vi "网分校准.vi"(8 "error in (no error)":errorcluster, 11 "keysight in":refnum<class "keysight.lvclass">) -> (0 "error out":errorcluster, 3 "keysight out":refnum<class "keysight.lvclass">)   [LabVIEW 2015, in "keysight.lvclass"]
uses:
  keysight.lvclass
  network_Global/Global.vi
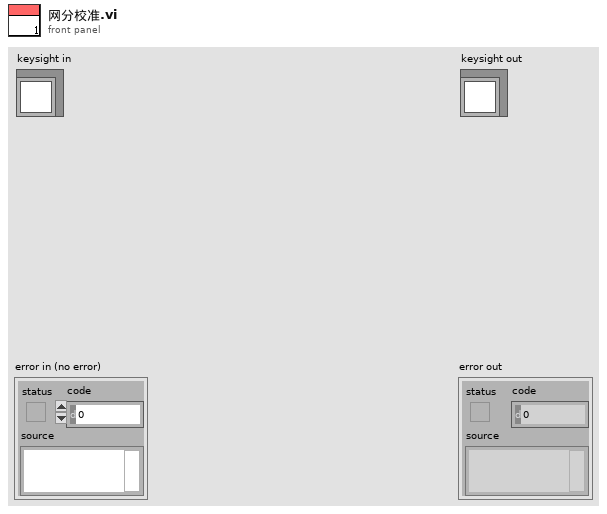
[diagram p1: front panel]
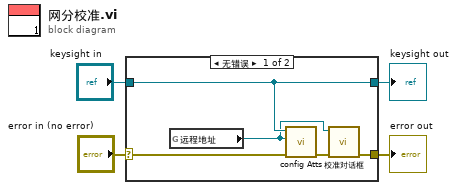
[diagram p0: block diagram]
diagram:
  n1 = case shown="无错误" "error in (no error)" {
    selector: "error in (no error)" -> [w6 w11]
    tunnel: "keysight in" -> [w9 w10]
    tunnel: [w9 w10] -> w2
    tunnel: [w5 w11] -> w1
    frame No Error {
      n2 = global read "Global.vi" "远程地址"() -> (w8:refnum<visa-resource-name>)
      n3 = call-dynamic "config Atts.vi"("error in (no error)"=w6, "VISA resource name"=w8, "keysight in"=w9) -> ("error out"=w7:errorcluster)  [unwired: 6 in, 2 out]
      n4 = call "校准对话框.vi"("error in (no error)"=w7, "VISA Refnum in"=w8) -> ("error out"=w5:errorcluster)  [unwired: 8 in, 1 out]
    }
    frame Error {
    }
  }
  "error out" <- w1
  "keysight out" <- w2
